vi "TEST - Array to VCluster.vi"(8 "error in (no error)":errorcluster) -> (0 "error out":errorcluster, 2 "pass":bool)   [LabVIEW 2020, in "test_openg_variant.lvlib"]
uses:
  test_openg_variant.lvlib
  <vilib>/addons/_JKI Toolkits/Caraya/classes/Assert/Assert True.vi
  source/library/openg_variant.lvlib
  <vilib>/addons/_JKI Toolkits/Caraya/classes/Test/Test.lvclass
  <vilib>/addons/_JKI Toolkits/Caraya/classes/Assert/Assert.lvclass
panel:
  out "Expected Result":T1
  out "Result":T1
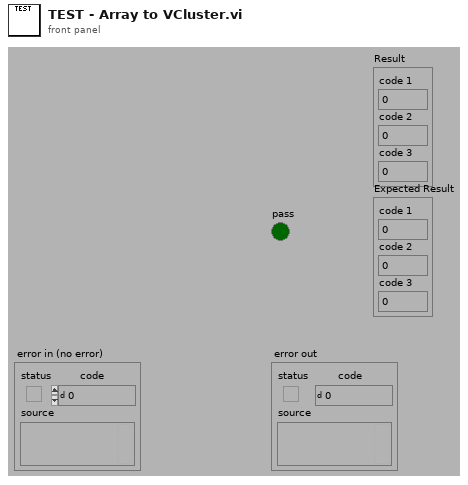
[diagram p1: front panel]
types:
  T1 = cluster{"code 1":i32, "code 2":i32, "code 3":i32}
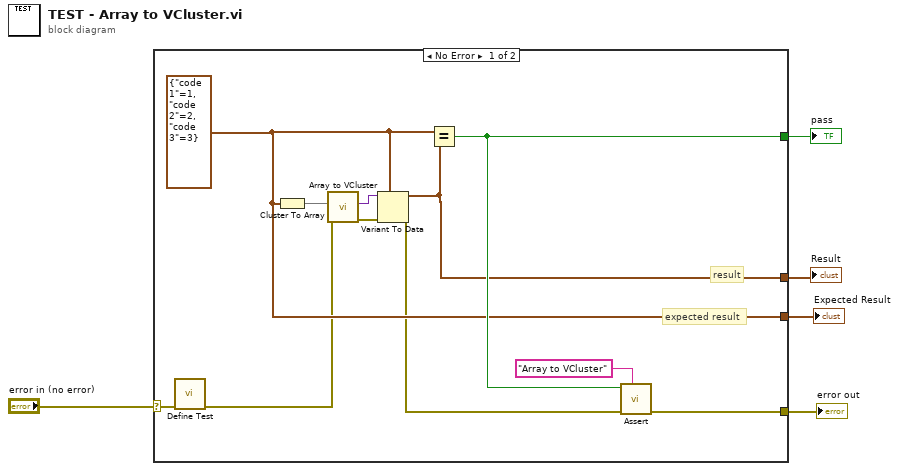
[diagram p0: block diagram]
diagram:
  n1 = case shown="No Error" "error in (no error)" {
    selector: "error in (no error)" -> [w9 w17]
    tunnel: [w13 _] -> w5
    tunnel: [w6 w17] -> w3
    tunnel: [w12 _] -> w2
    tunnel: [w11 _] -> w1
    frame No Error {
      w11 = T1 {"code 1"=1, "code 2"=2, "code 3"=3}
      # "result"
      # "expected result"
      n2 = call <vilib>:"Define Test.vi"("error in (no error)"=w9) -> ("error out"=w8:errorcluster)  [unwired: 9 in, 1 out]
      n3 = Cluster To Array(cluster=w11) -> (array=w16:i32[])
      n4 = call "Array to VCluster.vi"("error in (no error)"=w8, "Array"=w16) -> ("error out"=w14:errorcluster, "VCluster"=w15:variant)  [unwired: 8 in]
      n5 = Variant To Data(error in=w14, type=w11, Variant=w15) -> (data=w12:T1, error out=w7:errorcluster)
      n6 = Equal?(x=w11, y=w12) -> (x = y?=w13:bool)
      n7 = call-poly <vilib>:"Assert.vi"("Label"="Array to VCluster" ("Label (VI Title)"), "error in (no error)"=w7, "True?"=w13) -> ("error out"=w6:errorcluster)  [unwired: 7 in, 1 out]
    }
    frame Error {
    }
  }
  "pass" <- w5
  "error out" <- w3
  "Result" <- w2
  "Expected Result" <- w1
